vi "Expt2_MT QAM Transceiver_Student.vi"(5 "TX Filter":T2(ring)=enum."Raised Cosine", 7 "Eb/N0, dB":dbl(slide)=40.0 scale=0.0..100.0, 9 "Reset":bool=TRUE, 14 "?":T3(tab)=enum."Constellation (TX output)") -> (3 "QAM System Parameters":T6={"samples per symbol (16)"=16, "symbol map"=[]} {"symbol map" format="%.3f"}, 4 "Output Complex Waveform":cluster{"t0":dbl, "dt":dbl, "Values":cdb[]} {"Values" format="%.3f"; "dt" format="%^.2e"; "t0" format="%.4f"}, 6 "Transmitted Bits":i8[](array[numeric]), 8 "Received Bits":i8[](array[numeric]), 13 "Last Sync Found Index":dbl format="%.4f", 15 "Error Out":errorcluster)   [LabVIEW 2020]
doc: "This example demonstrates generation and analysis of QAM modulated signals. You can specify transmit filter parameters, Eb/No, and frequency offset. This example deomonstrates programming techniques for resetting the transmitter in cases where the receiver (demodulator) lock is lost. You can view the results of the demodulation on an eye diagram and perform measurements such as bit error rate."
uses:
  <vilib>/addons/Modulation/Digital/Support/Controls/QAM System Parameters.ctl
  <vilib>/addons/Modulation/Digital/Support/Common/Validators/mod_AWGN Validate.vi
  <vilib>/addons/Modulation/Analog/support/mod_Set Error Source.vi
  <vilib>/addons/Modulation/Digital/Impairments/subVIs/mod_createSeeds.vi
  <vilib>/addons/Modulation/Digital/Impairments/subVIs/mod_IQ Impairments Gain Imbalance.vi
  <vilib>/addons/Modulation/Digital/Impairments/subVIs/mod_IQ Impairments Quadrature Skew.vi
  <vilib>/addons/Modulation/Digital/Impairments/subVIs/mod_IQ Impairments Axis Shear.vi
  <vilib>/addons/Modulation/Digital/Impairments/subVIs/mod_IQ Impairments DC Offset.vi
  <vilib>/addons/Modulation/Digital/Impairments/subVIs/mod_IQ Impairments Frequency Offset.vi
  <vilib>/addons/Modulation/Digital/Support/Common/Validators/mod_Validate Samples Per Symbol.vi
  <vilib>/addons/Modulation/Analog/support/Validators/mod_Validate Complex Waveform.vi
  <vilib>/Analysis/5stat.llb/RMS.vi
  <vilib>/Analysis/5stat.llb/RMS (DBL).vi
  <vilib>/addons/Modulation/Digital/Support/Common/mod_Apply Frequency Offset.vi
  <vilib>/addons/Modulation/Analog/support/Validators/mod_WFErrorHandler.vi
  <vilib>/addons/Modulation/Digital/Support/Common/mod_Apply Frequency Offset (Internal).vi
  <vilib>/addons/Modulation/Digital/General/subVIs/mod_Generate Bits PN Sequence.vi
  <vilib>/Analysis/1siggen.llb/Gaussian White Noise (obs 90).vi
  <vilib>/addons/Modulation/Digital/Support/Common/Validators/mod_IQ Impairments Validate.vi
  <vilib>/addons/Modulation/Digital/Demodulation/MT EbN0 Calculation(QAM).vi
  <vilib>/addons/Modulation/Digital/Demodulation/MT Calculate BER After Trigger (PN Sequence).vi
  <vilib>/addons/Modulation/Digital/General/MT Format Eye Diagram (complex).vi
  <vilib>/addons/Modulation/niDMT.lvlib
panel:
  out "Estimated Eb/N0(dB)":dbl
  in  "Symbol Rate":dbl=1000000.0 step=1000.0 format="%.2p"
  out "Frequency Offset (Hz)":dbl format="%.2f"
  in  "Frequency Offset, Hz":dbl(slide) scale=-1000.0..1000.0
  out "Modulation Error Ratio (dB)":dbl format="%.2f"
  in  "# Message Symbols":i32=1000
  in  "M-QAM":T1(ring)=enum."16"
  out "Bit Error Rate":dbl format="%.4e"
  out "Rho":dbl format="%.4f"
  in  "stop":bool
  out "BER Trigger Found ?":bool
  out "Transmitted Symbols":T4(graph)={{"1/x"=0.0, 1e-06, [], 1}, []}
  in  "?":enum16{"I", "Q"}(ring)
  out "Eye Diagram":cluster{"t0":dbl, "dt":dbl, "Y":dbl[]}[](graph)
  in  "autoscale":bool
  out "TX Constellation":T5(graph)
  out "Received Symbols":T4(graph)={{"1/x"=0.0, 1e-06, [], 1}, []}
  in  "autoscale RX Constellation":bool
  out "RX Constellation":T5(graph)
  out "EVM per Symbol":dbl[](graph)
  # "Transmitted QAM Symbols"
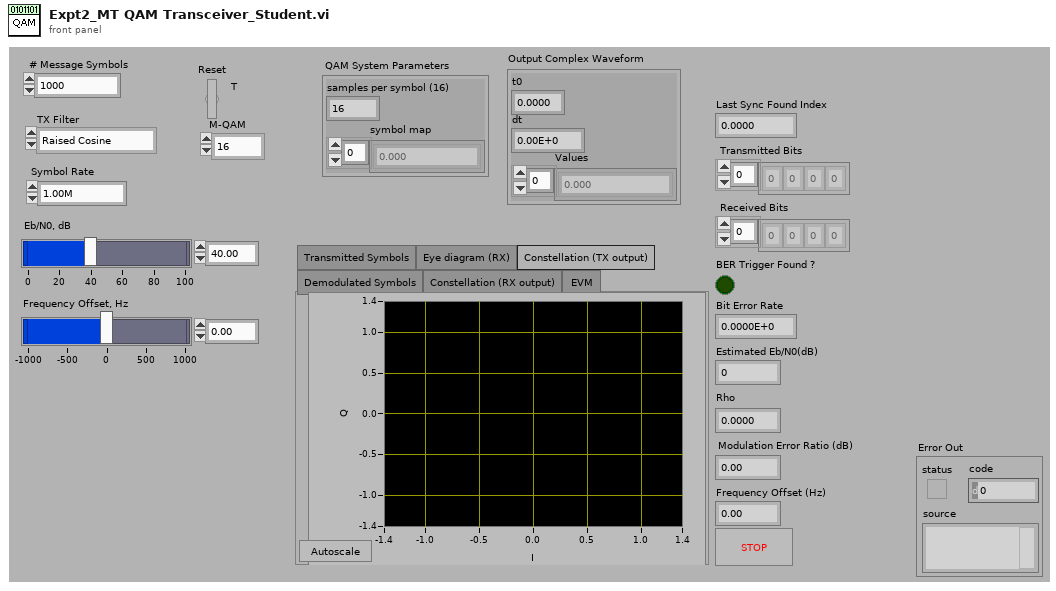
[diagram p1: front panel]
types:
  T1 = enum16{"4", "8", "16", "32", "64", "128", "256", "512", "1024", "2048", "4096"}
  T2 = enum16{"none", "Raised Cosine", "Root Raised Cos", "Gaussian"}
  T3 = enum32{"Transmitted Symbols", "Eye diagram (RX)", "Constellation (TX output)", "Demodulated Symbols", "Constellation (RX output)", "EVM "}
  T4 = cluster{cluster{"1/x":dbl, dbl, i8[], i32}, i32[][]}
  T5 = cluster{"Decimated Array":dbl[], "Decimated Array":dbl[]}[]
  T6 = typedef "niDMT.lvlib/QAM System Parameters.ctl" = cluster{"samples per symbol (16)":i32, "symbol map":cdb[]}
  T7 = cluster{"expected sync location (symbols)":i32, "sync sequence":cdb[], "sync location uncertainty (symbols)":i32, "sync indent (symbols)":i32}
  T8 = cluster{"TX Filter":enum16{"none", "Raised Cosine", "Root Raised Cos", "Gaussian"}, "filter parameter":dbl, "filter length":i32}
  T9 = cluster{"# Guard Bits":i32, "# Sync Bits":i32, "# Message Bits":i32, "PN sequence order":i32}
  T10 = typedef "niAMT.lvlib/Complex Data Waveform.ctl" = cluster{"t0":dbl, "dt":dbl, "Y":cdb[]}
  T11 = cluster{"Output Bit Stream":i8[], " # bits per symbol":i32, "Sync (Bits)":i8[], "Sync (Symbols)":cdb[], "pulse shaping filter coefficients":dbl[], "matched filter coefficients":dbl[], "QAM System Parameters":T6}
  T12 = cluster{"frequency offset (Hz)":dbl, "frequency drift (Hz)":dbl, "phase offset (deg)":dbl}
  T13 = cluster{"RMS measurement (%)":dbl, "peak measurement (%)":dbl, "peak symbol index":i32, "individual symbol measurements (%)":dbl[]}
  T14 = cluster{"constellation":dbl[], "oversampled data":dbl[]}[]
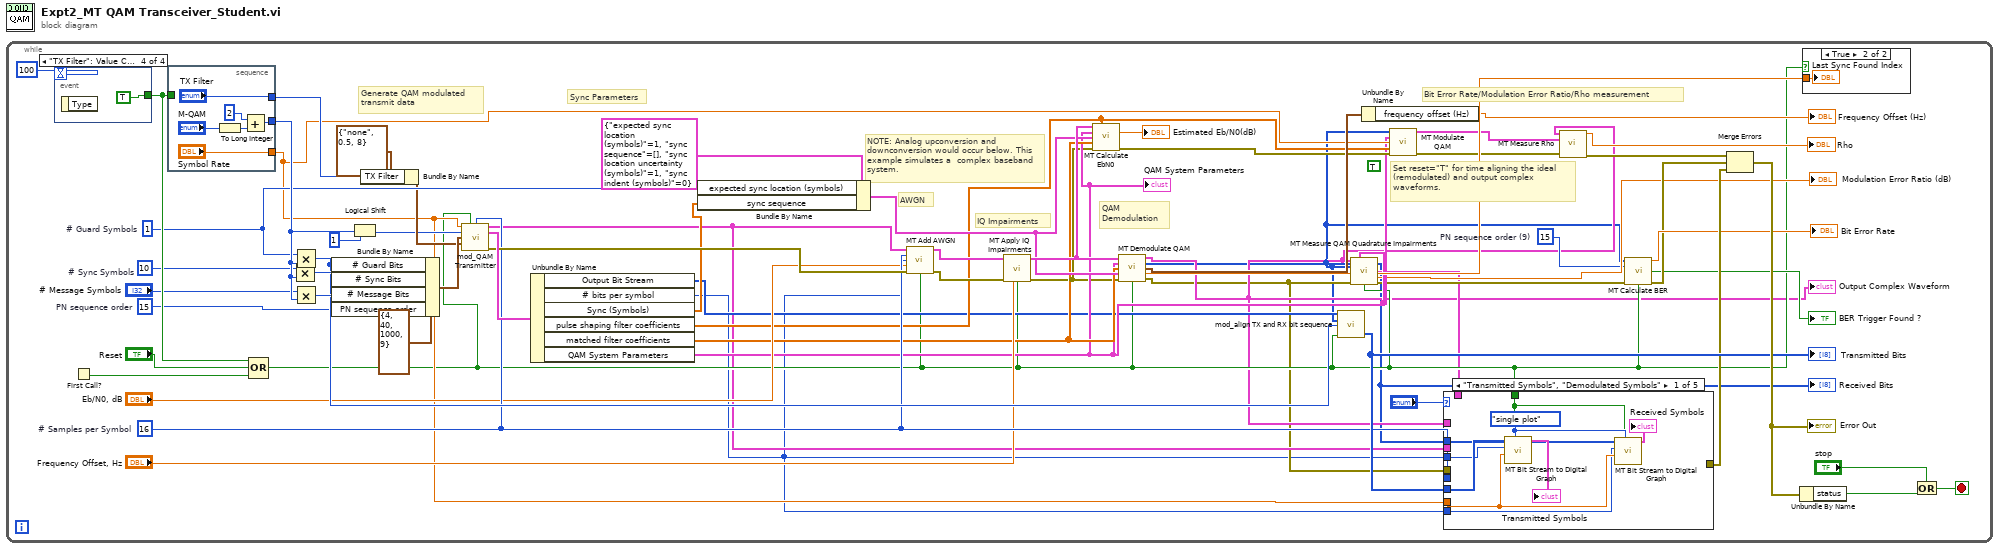
[diagram p0: block diagram]
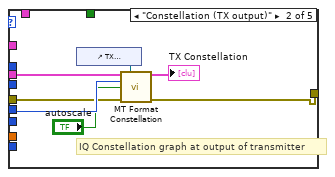
[diagram p2: hidden frame]
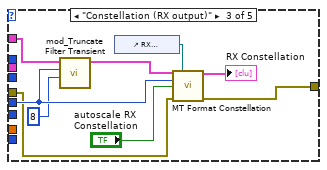
[diagram p3: hidden frame]
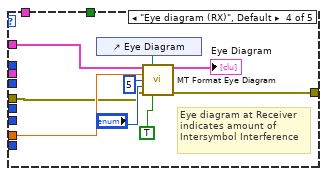
[diagram p4: hidden frame]
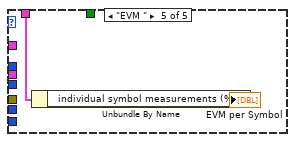
[diagram p5: hidden frame]
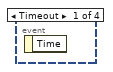
[diagram p7: hidden frame]
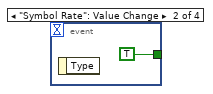
[diagram p8: hidden frame]
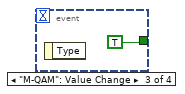
[diagram p9: hidden frame]
diagram:
  n1 = while {
    stop <- w63 stop-if-true
    w44 = 15  # PN sequence order
    w10 = 15  # PN sequence order (9)
    w36 = 16  # # Samples per Symbol
    w54 = 10  # # Sync Symbols
    w42 = 1  # # Guard Symbols
    (unwired) TRUE ("Reset? (T)")
    # "NOTE: Analog upconversion and downconversion would occur below. This example simulates a  complex baseband system."
    # "IQ Impairments"
    # "Bit Error Rate/Modulation Error Ratio/Rho measurement"
    # "Sync Parameters"
    # "Set reset=\"T\" for time aligning the ideal\n(remodulated) and output complex\nwaveforms."
    # "QAM \nDemodulation"
    # "Generate QAM modulated\ntransmit data"
    # "AWGN"
    n2 = event shown="[3] \"TX Filter\": Value Change" {
      selector: _ -> [_ _ _ _]
      dyn-events: _ -> [_ _ _ _]
      timeout: 100 -> [_ _ _ _]
      tunnel: [_ TRUE TRUE TRUE] -> w59
      event Timeout {
        n3 = event-data() -> ()  [unwired: 1 in, 1 out]
      }
      event "Symbol Rate": Value Change {
        n4 = event-data() -> ()  [unwired: 1 in, 1 out]
      }
      event "M-QAM": Value Change {
        n5 = event-data() -> ()  [unwired: 1 in, 1 out]
      }
      event "TX Filter": Value Change {
        n6 = event-data() -> ()  [unwired: 1 in, 1 out]
      }
    }
    n7 = First Call?() -> (First Call?: T/F=w60:bool)
    n8 = stacked-sequence {
      tunnel: w59 -> [_]
      tunnel: ["TX Filter"] -> w45
      tunnel: [w69] -> w55
      tunnel: ["Symbol Rate"] -> w18
      frame #0 {
        n9 = To Long Integer(number="M-QAM") -> (32bit integer=w68:i32)
        n10 = Add(x=2, y=w68) -> (x+y=w69:i32)
      }
    }
    n11 = Compound Arithmetic op=OR(w59, "Reset", w60) -> (w11:bool)
    n12 = Multiply(x=w54, y=w55) -> (x*y=w53:i32)
    n13 = Multiply(x=w42, y=w55) -> (x*y=w51:i32)
    n14 = Multiply(x="# Message Symbols", y=w55) -> (x*y=w52:i32)
    n15 = Bundle By Name(cluster=T9 {"# Guard Bits"=4, "# Sync Bits"=40, "# Message Bits"=1000, "PN sequence order"=9} ("Message"), "# Guard Bits"=w51, "# Sync Bits"=w53, "# Message Bits"=w52, "PN sequence order"=w44) -> (w40:T9)
    n16 = Logical Shift(y=w55, x=1) -> (x << y=w38:i32)
    n17 = Bundle By Name(cluster=T8 {"TX Filter"=enum."none", "filter parameter"=0.5, "filter length"=8} ("System Filter"), "TX Filter"=w45) -> (w39:T8)
    n18 = call <vilib>:"mod_QAM Transmitter.vi"("Symbol Rate, Hz"=w18, "Reset?"=w11, "# Samples per Symbol"=w36, "M-QAM"=w38, "Message"=w40, "System Filter"=w39) -> ("Output Complex Waveform"=w5:T10, "Signal Description"=w41:T11, "error out"=w37:errorcluster)  [unwired: 7 in]
    n19 = Unbundle By Name(w41) -> ("Output Bit Stream"=w12:i8[], "# bits per symbol"=w2:i32, "Sync (Symbols)"=w31:cdb[], "pulse shaping filter coefficients"=w17:dbl[], "matched filter coefficients"=w26:dbl[], "QAM System Parameters"=w16:T6)
    "QAM System Parameters" <- w16
    n20 = Bundle By Name(cluster=T7 {"expected sync location (symbols)"=1, "sync sequence"=[], "sync location uncertainty (symbols)"=1, "sync indent (symbols)"=0} ("synchronization parameters"), "expected sync location (symbols)"=w42, "sync sequence"=w31) -> (w27:T7)
    n21 = call <vilib>:"MT Add AWGN.vi"("input complex waveform"=w5, "samples per symbol (16)"=w36, "bits per symbol (1)"=w2, "Eb/N0 (10 dB)"="Eb/N0, dB", "error in (no error)"=w37, "reset? (T)"=w11) -> ("output complex waveform"=w34:T10, "error out"=w33:errorcluster)  [unwired: 7 in, 1 out]
    n22 = call <vilib>:"MT Apply IQ Impairments.vi"("input complex waveform"=w34, "error in (no error)"=w33, "frequency offset (Hz)"="Frequency Offset, Hz", "reset? (T)"=w11) -> ("output complex waveform"=w28:T10, "error out"=w8:errorcluster)  [unwired: 10 in]
    n23 = call-poly <vilib>:"MT Calculate EbN0.vi"("Recieved waveform"=w28, "pulse shaping filter coefficients"=w17, "QAM system parameters"=w16, "synchronization parameters"=w27, "matched filter coefficients"=w26, "error in (no error)"=w8) -> ("Eb/N0(dB)"=→"Estimated Eb/N0(dB)":dbl, "error out"=w19:errorcluster)  [unwired: 7 in, 1 out]
    n24 = call <vilib>:"MT Demodulate QAM.vi"("input complex waveform"=w28, "QAM system parameters"=w16, "matched filter coefficients"=w26, "synchronization parameters"=w27, "error in (no error)"=w8, "reset? (T)"=w11) -> ("recovered complex waveform"=w4:T10, "output bit stream"=w1:i8[], "measurements"=w30:T12, "sync found index (symbols)"=w29:dbl, "error out"=w3:errorcluster)  [unwired: 5 in]
    "Output Complex Waveform" <- w4
    "Received Bits" <- w1
    n25 = call <vilib>:"mod_align TX and RX bit sequence.vi"("TX Bit Sequence"=w12, "RX Bit Sequence"=w1, "# Bits removed"=w51, "Reset"=w11) -> ("Aligned array"=w50:i8[])  [unwired: 11 in]
    "Transmitted Bits" <- w50
    n26 = call <vilib>:"MT Measure QAM Quadrature Impairments.vi"("recovered complex waveform"=w4, "QAM system parameters"=w16, "input bit stream"=w1, "error in (no error)"=w3, "reset? (T)"=w11) -> ("EVM"=w6:T13, "modulation error ratio (dB)"=→"Modulation Error Ratio (dB)":dbl, "error out"=w9:errorcluster)  [unwired: 3 in, 5 out]
    n27 = Unbundle By Name(w30) -> ("frequency offset (Hz)"=→"Frequency Offset (Hz)":dbl)
    n28 = call <vilib>:"MT Modulate QAM.vi"("input bit stream"=w1, "QAM system parameters"=w16, "symbol rate (Hz)"=w18, "pulse shaping filter coefficients"=w17, "error in (no error)"=w19) -> ("output complex waveform"=w7:T10, "error out"=w20:errorcluster)  [unwired: 8 in, 1 out]
    n29 = case shown="\"Transmitted Symbols\", \"Demodulated Symbols\"" "?" {
      tunnel: w18 -> [w77 _ _ w104 _]
      tunnel: w50 -> [w76 _ _ _ _]
      tunnel: w36 -> [_ w85 w92 _ _]
      tunnel: [_ w84 w90 w100 _] -> w49
      tunnel: w11 -> [w75 _ _ _ _]
      tunnel: w6 -> [_ _ _ _ w106]
      tunnel: w5 -> [_ w82 _ _ _]
      tunnel: w4 -> [_ _ w89 w98 _]
      tunnel: w3 -> [_ w81 w88 w97 _]
      tunnel: w2 -> [w74 _ _ _ _]
      tunnel: w2 -> [w73 _ _ _ _]
      tunnel: w1 -> [w72 _ _ _ _]
      frame "Transmitted Symbols", "Demodulated Symbols" {
        w78 = enum16{"single plot", "plot per bit"}."single plot" ("Format")
        n30 = call <vilib>:"MT Bit Stream to Digital Graph.vi"("Reset (F)"=w75, "Format"=w78, "Symbol Rate (Hz)"=w77, "bits per symbol"=w73, "Bit Stream"=w76) -> ("Digital Waveform Graph"=→"Transmitted Symbols":T4)  [unwired: 6 in]
        n31 = call <vilib>:"MT Bit Stream to Digital Graph.vi"("Reset (F)"=w75, "Format"=w78, "Symbol Rate (Hz)"=w77, "bits per symbol"=w74, "Bit Stream"=w72) -> ("Digital Waveform Graph"=→"Received Symbols":T4)  [unwired: 6 in]
      }
      frame "Constellation (TX output)" {
        # "IQ Constellation graph at output of transmitter"
        n32 = control-ref of="TX Constellation"() -> (w86:refnum<vi>)
        n33 = call <vilib>:"MT Format Constellation.vi"("waveform"=w82, "constellation reference"=w86, "samples per symbol"=w85, "autoscale"="autoscale", "error in (no error)"=w81) -> ("constellation graph"=→"TX Constellation":T14, "error out"=w84:errorcluster)  [unwired: 9 in]
      }
      frame "Constellation (RX output)" {
        n34 = call <vilib>:"mod_Truncate Filter Transient.vi"("filter length (sym)"=8, "samples/symbol"=w92, "input complex waveform"=w89) -> ("output complex waveform"=w93:T10)  [unwired: 8 in]
        n35 = control-ref of="RX Constellation"() -> (w95:refnum<vi>)
        n36 = call <vilib>:"MT Format Constellation.vi"("waveform"=w93, "constellation reference"=w95, "samples per symbol"=w92, "autoscale"="autoscale RX Constellation", "error in (no error)"=w88) -> ("constellation graph"=→"RX Constellation":T14, "error out"=w90:errorcluster)  [unwired: 9 in]
      }
      frame "Eye diagram (RX)", Default {
        # "Eye diagram at Receiver\nindicates amount of\nIntersymbol Interference"
        n37 = control-ref of="Eye Diagram"() -> (w99:refnum<vi>)
        n38 = call-poly <vilib>:"MT Format Eye Diagram.vi"("waveform"=w98, "eye diagram reference"=w99, "symbol rate (Hz)"=w104, "eye length"=5, "I/Q (I)"="?", "error in (no error)"=w97, "autoscale"=TRUE) -> ("eye diagram"=→"Eye Diagram":cluster{"t0":dbl, "dt":dbl, "Y":dbl[]}[], "error out"=w100:errorcluster)  [unwired: 7 in]
      }
      frame "EVM " {
        n39 = Unbundle By Name(w106) -> ("individual symbol measurements (%)"=→"EVM per Symbol":dbl[])
      }
    }
    n40 = call <vilib>:"MT Measure Rho.vi"("received complex waveform"=w4, "ideal complex waveform"=w7, "error in (no error)"=w20) -> ("rho"=→"Rho":dbl, "error out"=w21:errorcluster)  [unwired: 11 in]
    n41 = call-poly <vilib>:"MT Calculate BER.vi"("input bit stream"=w1, "PN sequence order (9)"=w10, "error in (no error)"=w9, "reset? (T)"=w11) -> ("BER"=→"Bit Error Rate":dbl, "trigger found?"=→"BER Trigger Found ?":bool, "error out"=w22:errorcluster)  [unwired: 7 in, 2 out]
    n42 = Merge Errors(w21, w22, w49) -> (w58:errorcluster)
    "Error Out" <- w58
    n43 = Unbundle By Name(w58) -> ("status"=w64:bool)
    n44 = case shown="True" w11 {
      tunnel: w29 -> [_ w108]
      frame False {
      }
      frame True {
        "Last Sync Found Index" <- w108
      }
    }
    n45 = Or(x=w64, y="stop") -> (x .or. y?=w63:bool)
  }
